vi "3D map v2.vi"(0 "Map Data in":T1(array[cluster]), 1 "3d Points":cluster{"Data":sgl, "Data":sgl, "Data":sgl}[](array[cluster]), 2 "Sensor position":cluster{"X":sgl, "Y":sgl, "Z":sgl}, 3 "Kinect FOV (deg)":cluster{"Height":i32, "Width":i32}, 4 "Elevation Angle":i32, 5 "Sensor Yaw angle (deg)":dbl, 6 "Max distance":dbl, 7 "voxel length (in.)":dbl, 9 "Chunk length (voxel)":u8) -> (14 "Map Data out":T1(array[cluster]))   [LabVIEW 2014]
uses:
  <vilib>/Analysis/1siggen.llb/Ramp Pattern by Samples.vi
  <vilib>/Analysis/coordinate.llb/3D Coordinate Conversion (Array).vi
  <vilib>/Analysis/NI_AALPro.lvlib
  <vilib>/Analysis/NI_AALBase.lvlib
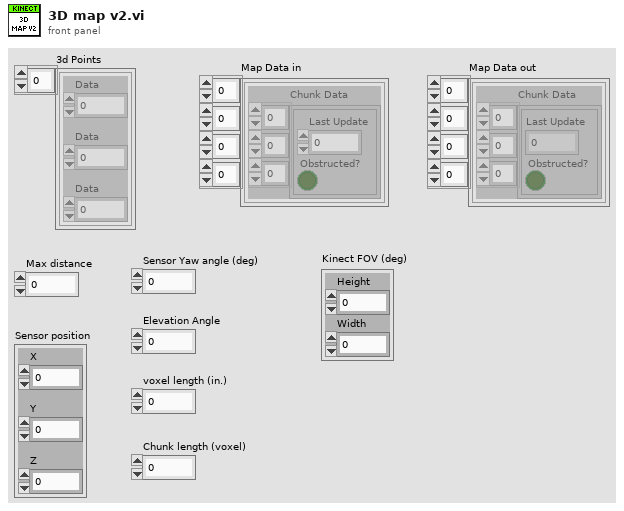
[diagram p1: front panel]
types:
  T1 = cluster{"Chunk Data":cluster{"Last Update":u32, "Obstructed?":bool}[][][]}[][][][]
  T2 = cluster{cluster{"Last Update":u32, bool}[][][]}[][][][]
  T3 = cluster{"Chunk Data":cluster{"Last Update":u32, "Obstructed?":bool}[][][]}
  T4 = cluster{"Last Update":u32, "Obstructed?":bool}[][][]
  T5 = cluster{"Numeric":dbl, "Numeric":dbl, "Numeric":dbl}[]
  T6 = cluster{"[0]":cluster{"Numeric":dbl, "Numeric":dbl, "Numeric":dbl}, "[1]":cluster{"Numeric":dbl, "Numeric":dbl, "Numeric":dbl}}
  T7 = cluster{"Numeric":dbl, "Numeric":dbl, "Numeric":dbl}
  T8 = cluster{"Numeric":bool, "Numeric":bool, "Numeric":bool}
  T9 = cluster{"voxel length (in.)":dbl, "Chunk length (voxel)":u8}
  T10 = enum16{"Voxel index", "Inches", "Voxel center (in)"}
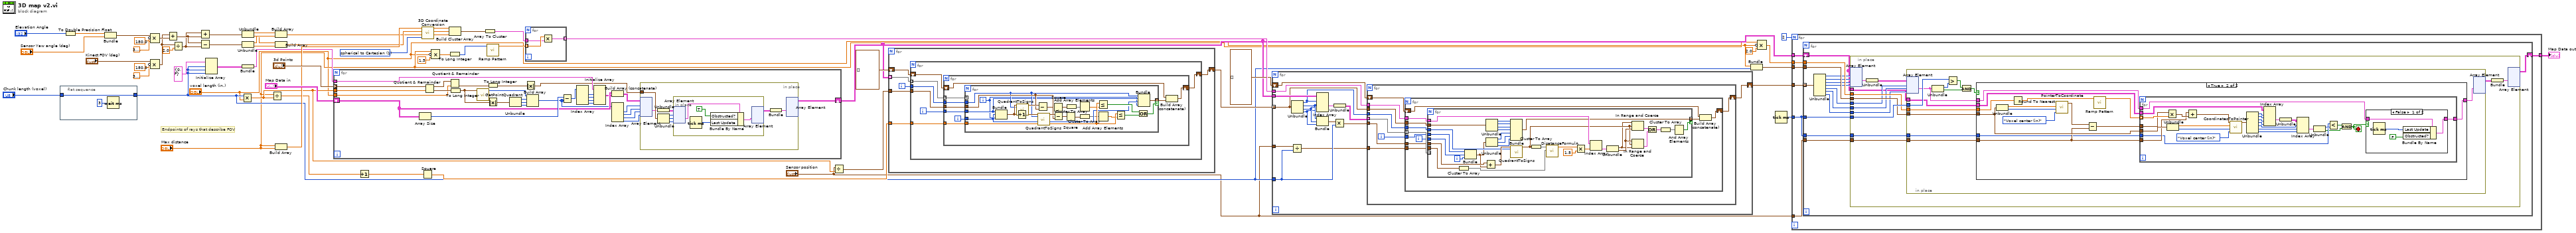
[diagram p0: block diagram]
diagram:
  w45 = u16 1 items=["Cartesian to spherical", "spherical to Cartesian", "Cartesian to cylindrical", "cylindrical to Cartesian", "spherical to cylindrical", "cylindrical to spherical"] ("conversion type")
  # "Endpoints of rays that describe FOV"
  n1 = flat-sequence {
    tunnel: "Chunk length (voxel)" -> [w62]
    tunnel: [w62] -> w10
    frame #0 {
      n2 = Wait (ms)(milliseconds to wait=u32 3) -> ()  [unwired: 1 out]
    }
  }
  n3 = To Double Precision Float(number="Elevation Angle") -> (double precision float=w52:dbl)
  n4 = Bundle(w52, "Sensor Yaw angle (deg)"="Sensor Yaw angle (deg)") -> (w53:cluster{dbl, "Sensor Yaw angle (deg)":dbl})  [unwired: 1 in]
  n5 = Compound Arithmetic op=MULTIPLY(w53, invert 180.0 ("value"), 3.141592653589793) -> (w50:cluster{dbl, "Sensor Yaw angle (deg)":dbl})
  n6 = Compound Arithmetic op=MULTIPLY("Kinect FOV (deg)", invert 180.0 ("value"), 3.141592653589793) -> (w48:cluster{"Height":dbl, "Width":dbl})
  n7 = Add(x=w48, y=w50) -> (x+y=w47:cluster{dbl, dbl})
  n8 = Divide(x=w48, y=2.0) -> (x/y=w46:cluster{"Height":dbl, "Width":dbl})
  n9 = Add(x=w46, y=w47) -> (x+y=w44:cluster{dbl, dbl})
  n10 = Subtract(x=w47, y=w46) -> (x-y=w43:cluster{dbl, dbl})
  n11 = Initialize Array(cluster{"Last Update":u32, bool} {"Last Update"=0, FALSE} ("Block Data"), w10, w10, w10) -> (w26:cluster{"Last Update":u32, bool}[][][])
  n12 = Multiply(x=w10, y="voxel length (in.)") -> (x*y=w23:dbl)
  n13 = Unbundle(w44) -> (w42:dbl, w39:dbl)
  n14 = Unbundle(w43) -> (w41:dbl, w40:dbl)
  n15 = Bundle(w26) -> (w25:cluster{cluster{"Last Update":u32, bool}[][][]})  [unwired: 1 in]
  n16 = Divide(x="Max distance", y=w23) -> (x/y=w29:dbl)
  n17 = Build Array(w42, w41) -> (w36:dbl[])
  n18 = Build Array(w39, w40) -> (w37:dbl[])
  n19 = Build Array("Max distance", "Max distance") -> (w38:dbl[])
  n20 = for {
    tunnel: "3d Points" -> [w92] mode=indexing
    tunnel: w23 -> [w91]
    tunnel: "voxel length (in.)" -> [w88]
    shift-right: [w86] -> w12
    shift-left: "Map Data in" -> [w75]
    tunnel: w25 -> [w68]
    n21 = Array Size(array=w75) -> (size(s)=w81:i32[])
    n22 = Quotient & Remainder(x=w92, y=w91) -> (x-y*floor(x/y)=w89:cluster{"Data":dbl, "Data":dbl, "Data":dbl}, floor(x/y)=w90:cluster{"Data":dbl, "Data":dbl, "Data":dbl})
    n23 = Quotient & Remainder(x=w89, y=w88) -> (floor(x/y)=w87:cluster{"Data":dbl, "Data":dbl, "Data":dbl})  [unwired: 1 out]
    n24 = To Long Integer(number=w90) -> (32bit integer=w65:cluster{"Data":i32, "Data":i32, "Data":i32})
    n25 = call "GetPointQuadrant.vi"("Point"=w65) -> ("Quadrant"=w85:i32)  [unwired: 4 in]
    n26 = To Long Integer(number=w87) -> (32bit integer=w64:cluster{"Data":i32, "Data":i32, "Data":i32})
    n27 = Absolute Value(x=w65) -> (abs(x)=w66:cluster{"Data":i32, "Data":i32, "Data":i32})
    n28 = Unbundle(w66) -> ("Data"=w84:i32, "Data"=w83:i32, "Data"=w82:i32)
    n29 = Absolute Value(x=w64) -> (abs(x)=w63:cluster{"Data":i32, "Data":i32, "Data":i32})
    n30 = Build Array(w85, w84, w83, w82) -> (w74:i32[])
    n31 = Subtract(x=w81, y=w74) -> (x-y=w80:i32[])
    n32 = Index Array(array=w80) -> (element #1=w79:i32, element #2=w78:i32, element #3=w77:i32, element #4=w76:i32)  [unwired: 4 in]
    n33 = Initialize Array(w68, w79, w78, w77, w76) -> (w67:T2)
    n34 = Build Array (concatenate)(w75, w67) -> (w73:T1)
    n35 = Index Array(array=w74) -> (element #1=w72:i32, element #2=w71:i32, element #3=w70:i32, element #4=w69:i32)  [unwired: 4 in]
    n36 = in-place {
      in-place-border: w63 -> [w100]
      n37 = in-place-array #1(w73, w72, w71, w70, w69) -> (w95:T3)
      n38 = Unbundle(w95) -> ("Chunk Data"=w94:T4)
      n39 = Unbundle(w100) -> ("Data"=w99:i32, "Data"=w98:i32, "Data"=w97:i32)
      n40 = in-place {
        n41 = in-place-array #2(w94, w99, w98, w97) -> (w103:cluster{"Last Update":u32, "Obstructed?":bool})
        n42 = Tick Count (ms)() -> (millisecond timer value=w104:u32)
        n43 = Bundle By Name(cluster=w103, "Obstructed?"=TRUE, "Last Update"=w104) -> (w102:cluster{"Last Update":u32, "Obstructed?":bool})
        n44 = in-place-array #2(w102) -> (w96:T4)  [unwired: 3 out]
      }
      n45 = Bundle("Chunk Data"=w96) -> (w93:T3)  [unwired: 1 in]
      n46 = in-place-array #1(w93) -> (w86:T1)  [unwired: 4 out]
    }
  }
  n47 = Increment(x=w29) -> (x+1=w28:dbl)
  n48 = Square(x=w28) -> (x^2=w34:dbl)
  n49 = call-poly <vilib>:"3D Coordinate Conversion.vi"("conversion type"=w45, "Axis 3"=w36, "Axis 2"=w37, "Axis 1"=w38) -> ("Axis 3 Out"=w30:dbl[], "Axis 2 Out"=w31:dbl[], "Axis 1 Out"=w32:dbl[])  [unwired: 4 in, 1 out]
  n50 = Compound Arithmetic op=MULTIPLY("Max distance", invert "voxel length (in.)", 1.5 ("value")) -> (w21:dbl)
  n51 = To Long Integer(number=w21) -> (32bit integer=w20:i32)
  n52 = Build Cluster Array(w32, w31, w30) -> (w18:T5)
  n53 = Array To Cluster(array=w18) -> (cluster=w17:T6)
  n54 = call-poly <vilib>:"Ramp Pattern.vi"("samples"=w20) -> ("Ramp Pattern"=w19:dbl[])  [unwired: 9 in, 1 out]
  n55 = for {
    tunnel: w19 -> [w107] mode=indexing
    tunnel: w17 -> [w106]
    tunnel: [w105] -> w15 mode=indexing
    n56 = Multiply(x=w107, y=w106) -> (x*y=w105:T6)
  }
  n57 = Divide(x="Sensor position", y=w23) -> (x/y=w35:cluster{"X":dbl, "Y":dbl, "Z":dbl})
  n58 = for {
    tunnel: w12 -> [w113] mode=indexing
    tunnel: w35 -> [w111]
    tunnel: w34 -> [w110]
    shift-right: [w109] -> w16
    shift-left: cluster{i32, i32, i32, i32}[] [] -> [w108]
    i -> [w112]
    n59 = for {
      tunnel: w113 -> [w120] mode=indexing
      tunnel: w112 -> [w119]
      tunnel: w111 -> [w118]
      tunnel: w110 -> [w117]
      shift-right: [w116] -> w109
      shift-left: w108 -> [w115]
      i -> [w114]
      n60 = for {
        tunnel: w120 -> [w129] mode=indexing
        tunnel: w119 -> [w128]
        tunnel: w118 -> [w127]
        tunnel: w117 -> [w126]
        shift-right: [w125] -> w116
        shift-left: w115 -> [w124]
        tunnel: w114 -> [w123]
        i -> [w122]
        n61 = for {
          tunnel: w129 -> [_] mode=indexing
          tunnel: w128 -> [w141]
          tunnel: w127 -> [w147]
          tunnel: w126 -> [w144]
          tunnel: w123 -> [w140]
          tunnel: w122 -> [w139]
          tunnel: [w137] -> w121 mode=indexing if=w130
          i -> [w138]
          n62 = Bundle(w140, w139, w138) -> (w150:cluster{i32, i32, i32})  [unwired: 1 in]
          n63 = Increment(x=w150) -> (x+1=w151:cluster{i32, i32, i32})
          n64 = call "QuadrantToSigns.vi"("Point"=w150, "Quadrant"=w141) -> ("Point Out"=w148:cluster{"X":sgl, "Y":sgl, "Z":sgl})  [unwired: 17 in]
          n65 = Subtract(x=w148, y=w147) -> (x-y=w146:cluster{"X":dbl, "Y":dbl, "Z":dbl})
          n66 = call "QuadrantToSigns.vi"("Point"=w151, "Quadrant"=w141) -> ("Point Out"=w149:cluster{"X":sgl, "Y":sgl, "Z":sgl})  [unwired: 17 in]
          n67 = Square(x=w146) -> (x^2=w136:cluster{"X":dbl, "Y":dbl, "Z":dbl})
          n68 = Subtract(x=w149, y=w147) -> (x-y=w145:cluster{"X":dbl, "Y":dbl, "Z":dbl})
          n69 = Square(x=w145) -> (x^2=w135:cluster{"X":dbl, "Y":dbl, "Z":dbl})
          n70 = Cluster To Array(cluster=w136) -> (array=w134:dbl[])
          n71 = Add Array Elements(numeric array=w134) -> (sum=w132:dbl)
          n72 = Cluster To Array(cluster=w135) -> (array=w133:dbl[])
          n73 = Less Or Equal?(x=w144, y=w132) -> (x <= y?=w142:bool)
          n74 = Add Array Elements(numeric array=w133) -> (sum=w131:dbl)
          n75 = Less Or Equal?(x=w144, y=w131) -> (x <= y?=w143:bool)
          n76 = Or(x=w142, y=w143) -> (x .or. y?=w130:bool)
          n77 = Bundle(w141, w140, w139, w138) -> (w137:cluster{i32, i32, i32, i32})  [unwired: 1 in]
        }
        n78 = Build Array (concatenate)(w124, w121) -> (w125:cluster{i32, i32, i32, i32}[])
      }
    }
  }
  n79 = for {
    tunnel: w16 -> [w154] mode=indexing
    tunnel: w12 -> [w167]
    tunnel: w15 -> [w161]
    tunnel: w10 -> [w157]
    tunnel: "Sensor position" -> [w158]
    shift-right: [w153] -> w13
    shift-left: cluster{i32, i32, i32, i32, i32, i32, i32}[] [] -> [w152]
    n80 = Divide(x=w158, y=w157) -> (x/y=w156:cluster{"X":sgl, "Y":sgl, "Z":sgl})
    n81 = Unbundle(w154) -> (w155:i32, w166:i32, w165:i32, w164:i32)
    n82 = Index Array(array=w167, index (dim 0)=w155, index (dim 1)=w166, index (dim 2)=w165, index (dim 3)=w164) -> (element=w163:T3)
    n83 = Bundle(w166, w165, w164) -> (w160:cluster{i32, i32, i32})  [unwired: 1 in]
    n84 = Multiply(x=w160, y=w157) -> (x*y=w159:cluster{i32, i32, i32})
    n85 = Unbundle(w163) -> ("Chunk Data"=w162:T4)
    n86 = for {
      tunnel: w162 -> [w176] mode=indexing
      tunnel: w159 -> [w174]
      tunnel: w161 -> [w173]
      tunnel: w156 -> [w172]
      tunnel: w155 -> [w171]
      tunnel: w154 -> [w170]
      shift-right: [w169] -> w153
      shift-left: w152 -> [w168]
      i -> [w175]
      n87 = for {
        tunnel: w176 -> [w187] mode=indexing
        tunnel: w175 -> [w186]
        tunnel: w174 -> [w184]
        tunnel: w173 -> [w183]
        tunnel: w172 -> [w182]
        tunnel: w171 -> [w181]
        tunnel: w170 -> [w180]
        shift-right: [w178] -> w169
        shift-left: w168 -> [w177]
        i -> [w185]
        n88 = for {
          tunnel: w187 -> [_] mode=indexing
          tunnel: w186 -> [w217]
          tunnel: w185 -> [w218]
          tunnel: w184 -> [w216]
          tunnel: w183 -> [w209]
          tunnel: w182 -> [w212]
          tunnel: w181 -> [w214]
          tunnel: w180 -> [w199]
          tunnel: [w191] -> w179 mode=indexing if=w190
          i -> [w219]
          n89 = Cluster To Array(cluster=w212) -> (array=w211:sgl[])
          n90 = Bundle(w217, w218, w219) -> (w200:cluster{i32, i32, i32})  [unwired: 1 in]
          n91 = Add(x=w216, y=w200) -> (x+y=w215:cluster{i32, i32, i32})
          n92 = Unbundle(w199) -> (w198:i32, w197:i32, w196:i32, w195:i32)
          n93 = Unbundle(w200) -> (w194:i32, w193:i32, w192:i32)
          n94 = Bundle(w198, w197, w196, w195, w194, w193, w192) -> (w191:cluster{i32, i32, i32, i32, i32, i32, i32})  [unwired: 1 in]
          n95 = call "QuadrantToSigns.vi"("Point"=w215, "Quadrant"=w214) -> ("Point Out"=w206:cluster{"X":sgl, "Y":sgl, "Z":sgl})  [unwired: 17 in]
          n96 = Cluster To Array(cluster=w206) -> (array=w213:sgl[])
          n97 = call "DisatanceFormulA.vi"("B"=w211, "A"=w213) -> ("Distance"=w189:dbl)  [unwired: 9 in]
          n98 = Multiply(x=w189, y=1.5) -> (x*y=w210:dbl)
          n99 = Index Array(array=w209, index=w210) -> (element=w208:T6)
          n100 = Unbundle(w208) -> ("[0]"=w205:T7, "[1]"=w207:T7)
          n101 = In Range and Coerce(upper limit=w205, x=w206, lower limit=w207) -> (In Range?=w203:T8)  [unwired: 1 out]
          n102 = In Range and Coerce(upper limit=w207, x=w206, lower limit=w205) -> (In Range?=w204:T8)  [unwired: 1 out]
          n103 = Or(x=w203, y=w204) -> (x .or. y?=w202:T8)
          n104 = Cluster To Array(cluster=w202) -> (array=w201:bool[])
          n105 = And Array Elements(Boolean array=w201) -> (logical AND=w190:bool)
        }
        n106 = Build Array (concatenate)(w177, w179) -> (w178:cluster{i32, i32, i32, i32, i32, i32, i32}[])
      }
    }
  }
  n107 = Bundle("voxel length (in.)"="voxel length (in.)", "Chunk length (voxel)"=w10) -> (w9:T9)  [unwired: 1 in]
  n108 = Compound Arithmetic op=MULTIPLY("Max distance", invert "voxel length (in.)", 2.0 ("value")) -> (w5:dbl)
  n109 = Tick Count (ms)() -> (millisecond timer value=w3:u32)
  n110 = for {
    N: 2 -> [_]
    tunnel: w13 -> [w226]
    tunnel: w12 -> [w225]
    tunnel: w9 -> [w224]
    tunnel: "Sensor position" -> [w223]
    tunnel: w5 -> [w222]
    tunnel: w3 -> [w221]
    tunnel: [w220] -> w1
    n111 = for {
      tunnel: w226 -> [w240] mode=indexing
      tunnel: w221 -> [w241]
      shift-right: [w229] -> w220
      shift-left: w225 -> [w228]
      tunnel: w224 -> [w238]
      tunnel: w223 -> [w239]
      tunnel: w222 -> [w237]
      tunnel: w221 -> [w227]
      n112 = Unbundle(w240) -> (w236:i32, w235:i32, w234:i32, w233:i32, w232:i32, w231:i32, w230:i32)
      n113 = in-place {
        in-place-border: w241 -> [w254]
        in-place-border: w239 -> [w253]
        in-place-border: w238 -> [w252]
        in-place-border: w237 -> [w251]
        in-place-border: w232 -> [w248]
        in-place-border: w231 -> [w247]
        in-place-border: w230 -> [w246]
        in-place-border: w228 -> [w243]
        in-place-border: w227 -> [w242]
        n114 = in-place-array #3(w228, w236, w235, w234, w233) -> (w250:T3)
        n115 = Unbundle(w250) -> ("Chunk Data"=w249:T4)
        n116 = in-place {
          in-place-border: w254 -> [w266]
          in-place-border: w253 -> [w263]
          in-place-border: w252 -> [w262]
          in-place-border: w251 -> [w261]
          in-place-border: w243 -> [w258]
          in-place-border: w242 -> [w257]
          n117 = in-place-array #4(w249, w248, w247, w246) -> (w256:cluster{"Last Update":u32, "Obstructed?":bool})
          n118 = Unbundle(w256) -> ("Last Update"=w260:u32, "Obstructed?"=w259:bool)
          n119 = Greater?(x=w266, y=w260) -> (0:w265:bool)
          n120 = And(x=w265, y=w259) -> (x .and. y?=w264:bool)
          n121 = case shown="True" w264 {
            tunnel: w263 -> [_ w272]
            tunnel: w262 -> [_ w273]
            tunnel: w261 -> [_ w276]
            tunnel: w258 -> [_ w271]
            tunnel: w257 -> [_ w270]
            tunnel: w256 -> [w267 w269]
            tunnel: [w267 w268] -> w255
            frame False {
            }
            frame True {
              n122 = Unbundle(w273) -> ("voxel length (in.)"=w280:dbl, "Chunk length (voxel)"=w279:u8)
              n123 = Round To Nearest(number=w276) -> (nearest integer value=w277:dbl)
              n124 = call "PointerToCoordinate.vi"("Return Type"=T10."Voxel center (in)", "Chunk length"=w279, "Voxel length"=w280) -> ("Coordinates"=w278:cluster{dbl, dbl, dbl})  [unwired: 8 in]
              n125 = Subtract(x=w278, y=w272) -> (x-y=w274:cluster{dbl, dbl, dbl})
              n126 = call-poly <vilib>:"Ramp Pattern.vi"("samples"=w277) -> ("Ramp Pattern"=w275:dbl[])  [unwired: 9 in, 1 out]
              n127 = for {
                tunnel: w275 -> [w305] mode=indexing
                tunnel: w274 -> [w304]
                tunnel: w273 -> [w307]
                tunnel: w272 -> [w302]
                tunnel: w271 -> [w298]
                tunnel: w270 -> [w287]
                tunnel: w269 -> [w284]
                tunnel: [w282] -> w268
                stop <- w283 stop-if-true
                n128 = Multiply(x=w304, y=w305) -> (x*y=w303:cluster{dbl, dbl, dbl})
                n129 = Unbundle(w307) -> ("voxel length (in.)"=w309:dbl, "Chunk length (voxel)"=w308:u8)
                n130 = Add(x=w302, y=w303) -> (x+y=w301:cluster{dbl, dbl, dbl})
                n131 = call "CoordinatesToPointer.vi"("Input Type"=T10."Voxel center (in)", "Chunk length"=w308, "Voxel length"=w309, "Coordinates"=w301) -> ("Voxel pointer"=w300:cluster{i32, i32, i32, i32, i32, i32, i32})  [unwired: 7 in]
                n132 = Unbundle(w300) -> (w299:i32, w297:i32, w296:i32, w295:i32, w292:i32, w291:i32, w290:i32)
                n133 = Index Array(array=w298, index (dim 0)=w299, index (dim 1)=w297, index (dim 2)=w296, index (dim 3)=w295) -> (element=w294:T3)
                n134 = Unbundle(w294) -> ("Chunk Data"=w293:T4)
                n135 = Index Array(array=w293, index (dim 0)=w292, index (dim 1)=w291, index (dim 2)=w290) -> (element=w289:cluster{"Last Update":u32, "Obstructed?":bool})
                n136 = Unbundle(w289) -> ("Last Update"=w288:u32, "Obstructed?"=w285:bool)
                n137 = Less?(x=w287, y=w288) -> (x < y?=w286:bool)
                n138 = And(x=w286, y=w285) -> (x .and. y?=w283:bool)
                n139 = case shown="False" w283 {
                  tunnel: w284 -> [w313 w314]
                  tunnel: [w312 w314] -> w282
                  frame False {
                    n140 = Tick Count (ms)() -> (millisecond timer value=w311:u32)
                    n141 = Bundle By Name(cluster=w313, "Last Update"=w311, "Obstructed?"=FALSE) -> (w312:cluster{"Last Update":u32, "Obstructed?":bool})
                  }
                  frame True {
                  }
                }
              }
            }
          }
          n142 = in-place-array #4(w255) -> (w245:T4)  [unwired: 3 out]
        }
        n143 = Bundle("Chunk Data"=w245) -> (w244:T3)  [unwired: 1 in]
        n144 = in-place-array #3(w244) -> (w229:T1)  [unwired: 4 out]
      }
    }
  }
  "Map Data out" <- w1
